vi "m10.wf.multipleOf2.vi"(0 "Waveform In":waveform(dbl), 11 "error in (no error)":errorcluster) -> (4 "Waveform Out":waveform(dbl), 15 "error out":errorcluster)   [LabVIEW 2009]
uses:
  <vilib>/Waveform/WDTOps.llb/WDT Number of Waveform Samples DBL.vi
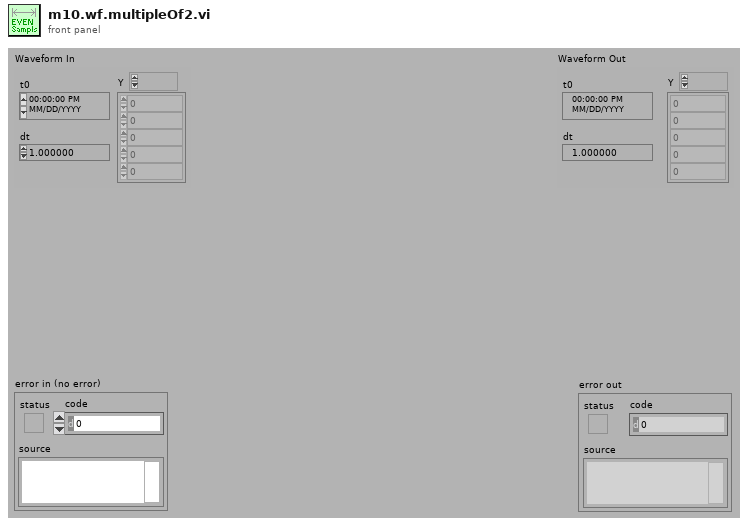
[diagram p1: front panel]
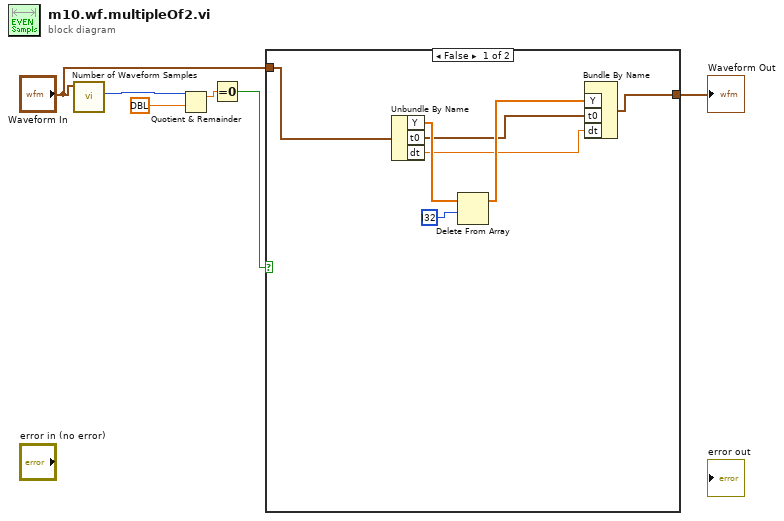
[diagram p0: block diagram]
diagram:
  n1 = call-poly <vilib>:"Number of Waveform Samples.vi"("waveform in"="Waveform In") -> ("number of samples"=w1:i32)  [unwired: 8 in, 2 out]
  n2 = Quotient & Remainder(x=w1, y=dbl ?) -> (x-y*floor(x/y)=w5:dbl)  [unwired: 1 out]
  n3 = Equal To 0?(x=w5) -> (x = 0?=w4:bool)
  n4 = case shown="False" w4 {
    tunnel: "Waveform In" -> [w11 w14]
    tunnel: [w13 w14] -> w3
    frame #0 {
      n5 = Unbundle By Name(w11) -> ("Y"=w10:dbl[], "t0"=w8:timestamp, "dt"=w7:dbl)
      n6 = Delete From Array(array=w10, length=i32 ?) -> (array with subset deleted=w9:dbl[])  [unwired: 1 in, 1 out]
      n7 = Bundle By Name("Y"=w9, "t0"=w8, "dt"=w7) -> (w13:waveform(dbl))  [unwired: 1 in]
    }
    frame #1 {
    }
  }
  "Waveform Out" <- w3
